vi "Read Key.vi"(8 "Error In":errorcluster, 11 "UnescapedVariable In":refnum<class "UnescapedVariable.lvclass">) -> (0 "Error Out":errorcluster, 2 "Key":string, 3 "UnescapedVariable Out":refnum<class "UnescapedVariable.lvclass">)   [LabVIEW 2017, in "Mustache.lvlib" / "Tokens.lvlib" / "UnescapedVariable.lvclass"]
uses:
  UnescapedVariable.lvclass
  UnescapedVariable.lvclass/UnescapedVariable.ctl
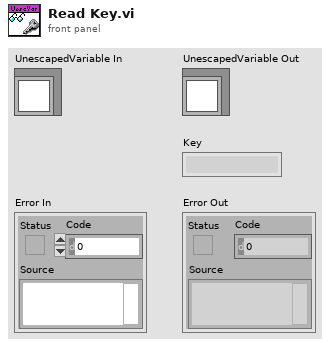
[diagram p1: front panel]
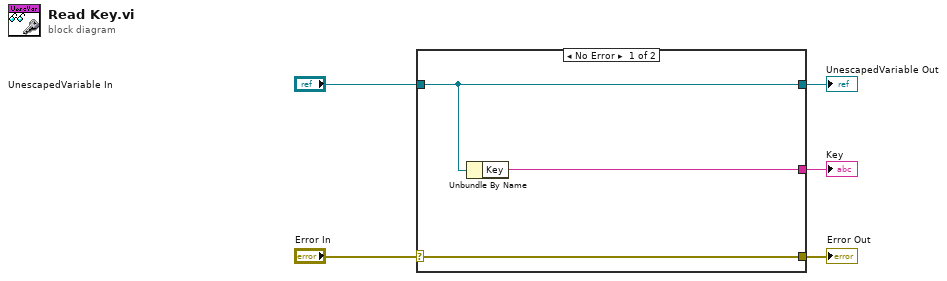
[diagram p0: block diagram]
diagram:
  n1 = case shown="No Error" "Error In" {
    selector: "Error In" -> [w8 w9]
    tunnel: [w8 w9] -> w4
    tunnel: [w7 w10] -> w2
    tunnel: "UnescapedVariable In" -> [w7 w10]
    tunnel: [w6 _] -> w1
    frame No Error {
      n2 = Unbundle By Name(w7) -> ("Key"=w6:string)
    }
    frame Error {
    }
  }
  "Error Out" <- w4
  "UnescapedVariable Out" <- w2
  "Key" <- w1
